vi "AprilTag Tag Familys string AE.vi"(11 "Tag Familys":string[](array[string])) -> (3 "Tag Familys String":string)   [LabVIEW 2025]
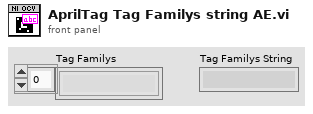
[diagram p1: front panel]
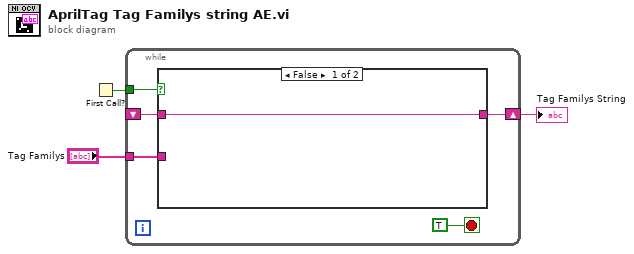
[diagram p0: block diagram]
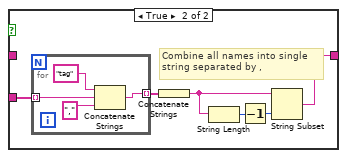
[diagram p2: hidden frame]
diagram:
  n1 = First Call?() -> (First Call?: T/F=w2:bool)
  n2 = while {
    tunnel: "Tag Familys" -> [w8]
    shift-right: [w6] -> w1
    shift-left: _ -> [w5]
    tunnel: w2 -> [w7]
    stop <- TRUE stop-if-true
    n3 = case shown="False" w7 {
      tunnel: [w9 w12] -> w6
      tunnel: w8 -> [_ w10]
      tunnel: w5 -> [w9 _]
      frame False {
      }
      frame True {
        # "Combine all names into single\nstring separated by ,"
        n4 = for {
          tunnel: w10 -> [w17] mode=indexing
          tunnel: [w18] -> w11 mode=indexing
          n5 = Concatenate Strings("tag" ("string"), w17, "," ("string")) -> (w18:string)
        }
        n6 = Concatenate Strings(w11) -> (w13:string)
        n7 = String Length(string=w13) -> (length=w14:i32)
        n8 = Decrement(x=w14) -> (x-1=w15:i32)
        n9 = String Subset(string=w13, length (rest)=w15) -> (substring=w12:string)  [unwired: 1 in]
      }
    }
  }
  "Tag Familys String" <- w1
